vi "Get model data.vi"(8 "error in (no error)":errorcluster, 11 "CMD_Str":string="select ModelNo from BSJRecord") -> (0 "error out":errorcluster, 2 "Model Names":string[](array[string]))   [LabVIEW 2013]
uses:
  <vilib>/addons/database/Connection.llb/DB Tools Open Connec (String).vi
  <vilib>/addons/database/Connection.llb/Conn Execute.vi
  <vilib>/addons/database/Recordset.llb/Rec Fetch Recordset Data (R).vi
  <vilib>/addons/database/Recordset.llb/Rec Destroy - Connection.vi
  <vilib>/addons/database/NI_Database_API.lvlib
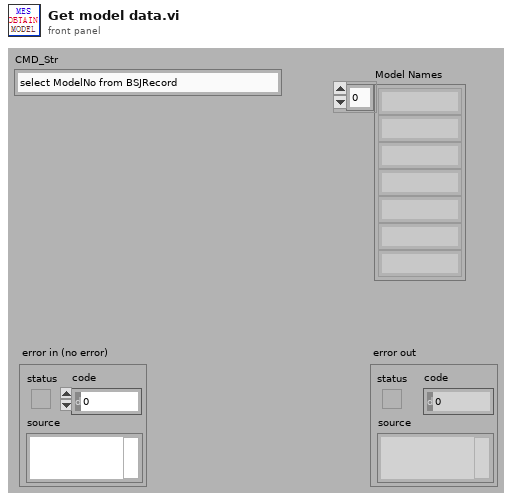
[diagram p1: front panel]
types:
  T1 = typedef "NI_Database_API.lvlib/Conn ObjectReference.ctl" = refnum<k1>
  T2 = typedef "NI_Database_API.lvlib/Rec ObjectReference.ctl" = refnum<k1>
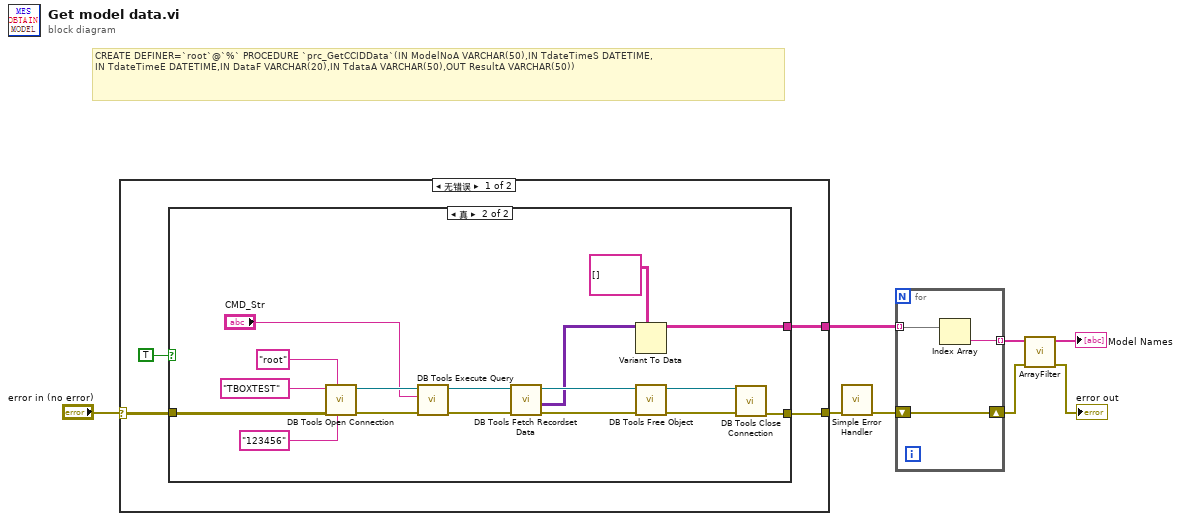
[diagram p0: block diagram]
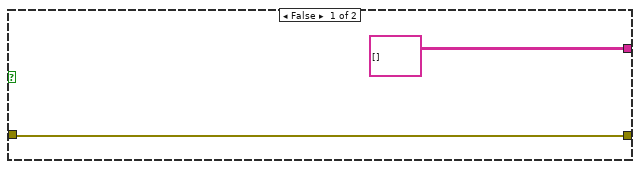
[diagram p2: hidden frame]
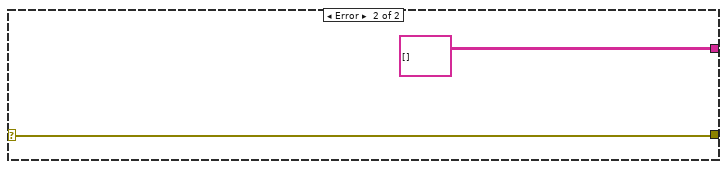
[diagram p3: hidden frame]
diagram:
  # "CREATE DEFINER=`root`@`%` PROCEDURE `prc_GetCCIDData`(IN ModelNoA VARCHAR(50),IN TdateTimeS DATETIME,\nIN TdateTimeE DATETIME,IN DataF VARCHAR(20),IN TdataA VARCHAR(50),OUT ResultA VARCHAR(50))"
  n1 = case shown="无错误" "error in (no error)" {
    selector: "error in (no error)" -> [w10 w33]
    tunnel: [w12 w33] -> w8
    tunnel: [w11 string[][] []] -> w6
    frame No Error {
      n2 = case shown="真" TRUE {
        tunnel: [w14 w25] -> w12
        tunnel: [string[][] [] w18] -> w11
        tunnel: w10 -> [w14 w17]
        frame False {
        }
        frame True {
          n3 = call-poly <vilib>:"DB Tools Open Connection.vi"("password"="123456", "userID"="root", "error in (no error)"=w17, "connection information"="TBOXTEST") -> ("error out"=w29:errorcluster, "connection reference"=w28:T1)  [unwired: 4 in]
          n4 = call-poly <vilib>:"DB Tools Execute Query.vi"("error in (no error)"=w29, "SQL query"="CMD_Str", "connection reference"=w28) -> ("error out"=w26:errorcluster, "recordset reference"=w27:T2)  [unwired: 5 in]
          n5 = call-poly <vilib>:"DB Tools Fetch Recordset Data.vi"("error in (no error)"=w26, "recordset reference"=w27) -> ("error out"=w24:errorcluster, "recordset data"=w20:variant[][], "recordset reference out"=w23:T2)  [unwired: 3 in]
          n6 = Variant To Data(type=string[][] [], Variant=w20) -> (data=w18:string[][])  [unwired: 1 in, 1 out]
          n7 = call-poly <vilib>:"DB Tools Free Object.vi"("error in (no error)"=w24, "recordset reference"=w23) -> ("error out"=w22:errorcluster, "connection reference"=w21:T1)  [unwired: 8 in]
          n8 = call <vilib>:"DB Tools Close Connection.vi"("error in (no error)"=w22, "connection reference"=w21) -> ("error out"=w25:errorcluster)  [unwired: 5 in]
        }
      }
    }
    frame Error {
    }
  }
  n9 = call <vilib>:"Simple Error Handler.vi"("error in (no error)"=w8) -> ("error out"=w5:errorcluster)  [unwired: 4 in, 4 out]
  n10 = for {
    tunnel: w6 -> [w35] mode=indexing
    shift-right: [w36] -> w2
    shift-left: w5 -> [w36]
    tunnel: [w34] -> w4 mode=indexing
    n11 = Index Array(array=w35) -> (element=w34:string)  [unwired: 1 in]
  }
  n12 = call "ArrayFilter.vi"("error in"=w2, "ArrayIn"=w4) -> ("error out"=→"error out":errorcluster, "ArrayOut"=→"Model Names":string[])  [unwired: 8 in]
